vi "get Data Element.vi"(0 "LVx - Template Command in":refnum<class "REx - NART - Load DUT.lvclass">, 11 "error in (no error)":errorcluster) -> (4 "LVx - Template Command out":refnum<class "REx - NART - Load DUT.lvclass">, 6 "Device Config":T1={"Device Type"=-1, "Device Template"=2, "Cal Mem Type"=0, "Cal Mem Size"=0} {"Cal Mem Size" items=["automatic"=0, "1K"=1024, "2K"=2048, "4K"=4096, "8K"=8192]; "Cal Mem Type" items=["none"=4, "auto"=0, "flash"=1, "eeprom"=2, "otp"=3]; "Device Template" items=["ar938x/9x"=2, "HB112"=3, "HB116"=4, "XB112"=5, "XB113"=6, "XB114"=7, "TB417"=8, "AP111"=9, "AP121"=10, "AR9330"=11]; "Device Type" items=["Default"=-1, "Osprey"=48, "Wasp"=49]}, 15 "error out":errorcluster)   [LabVIEW 2011, in "ART2 Test Panel.lvlib" / "REx - NART - Load DUT.lvclass"]
uses:
  REx - NART - Load DUT.lvclass
  Components/ART2.llb/NART/Controls/Load Config.ctl
  Components/ART2.llb/NART/Controls/NART Device Type.ctl
  Components/ART2.llb/NART/Controls/Preferred Starting Templates.ctl
  Components/ART2.llb/NART/Controls/Cal Data Memory Type.ctl
  Components/ART2.llb/NART/Controls/Calibration Memory Size.ctl
  REx - NART - Load DUT.lvclass/REx - NART - Load DUT.ctl
  ART2 Test Panel.lvlib
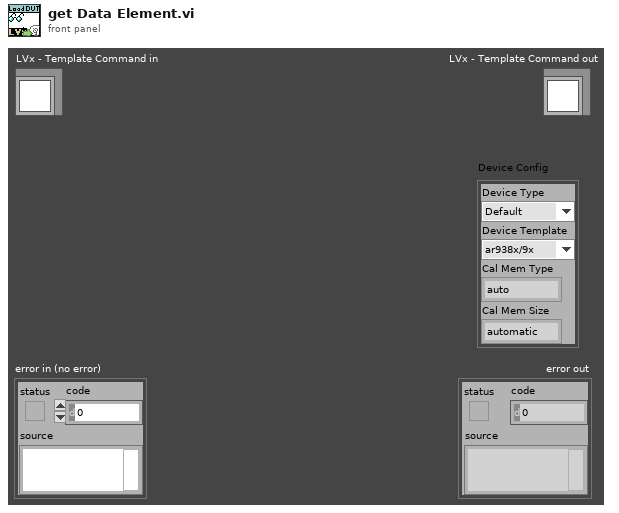
[diagram p1: front panel]
types:
  T1 = typedef "ART2 Test Panel.lvlib/Load Config.ctl" = cluster{"Device Type":T2, "Device Template":T3, "Cal Mem Type":T4, "Cal Mem Size":T5}
  T2 = typedef "ART2 Test Panel.lvlib/NART Device Type.ctl" = i32
  T3 = typedef "ART2 Test Panel.lvlib/Preferred Starting Templates.ctl" = i32
  T4 = typedef "ART2 Test Panel.lvlib/Cal Data Memory Type.ctl" = i32
  T5 = typedef "ART2 Test Panel.lvlib/Calibration Memory Size.ctl" = i32
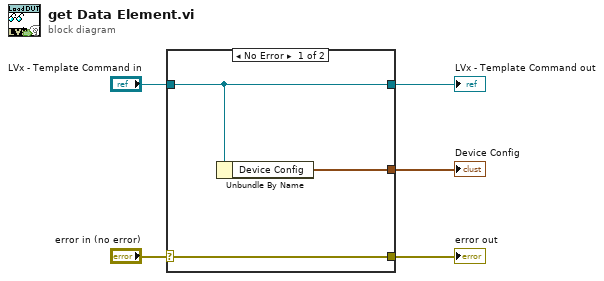
[diagram p0: block diagram]
diagram:
  n1 = case shown="No Error" "error in (no error)" {
    selector: "error in (no error)" -> [w8 w9]
    tunnel: [w8 w9] -> w4
    tunnel: [w6 w10] -> w2
    tunnel: "LVx - Template Command in" -> [w6 w10]
    tunnel: [w7 _] -> w1
    frame No Error {
      n2 = Unbundle By Name(w6) -> ("Device Config"=w7:T1)
    }
    frame Error {
    }
  }
  "error out" <- w4
  "LVx - Template Command out" <- w2
  "Device Config" <- w1
